vi "GV PreframeclockDelayed.vi"() -> ()   [LabVIEW 2017]
panel:
  out "PreframeclockDelayed":bool
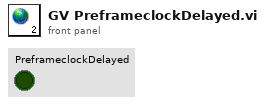
[diagram p1: front panel]
diagram:
